vi "Core.vi"(8 "error in (no error)":errorcluster, 10 "Actor in":refnum<class "Actor.lvclass">, 11 "Reorder Driver Aliases Msg in":refnum<class "Reorder Driver Aliases Msg.lvclass">) -> (0 "error out":errorcluster, 1 "Data":refnum<class "Data.lvclass">, 2 "Actor out":refnum<class "Actor.lvclass">, 3 "Reorder Driver Aliases Msg out":refnum<class "Reorder Driver Aliases Msg.lvclass">)   [LabVIEW 2020, in "Instrument Handler.lvlib" / "Reorder Driver Aliases Msg.lvclass"]
doc: "Core of the Reponse Msg. Put the active code here.\n\nThis implementation reorders Alias' on the Instrument Handler. On a succesfull operation a TRUE is returned in a generic Boolean data class."
uses:
  Reorder Driver Aliases Msg.lvclass
  PPL/HDH.Data.Generic.lvlibp/Data.lvclass
  PPL/HDH.Actor Framework.Core.Actor.lvlibp/1abvi3w/vi.lib/ActorFramework/Actor/Actor.lvclass
  Instrument Handler/Instrument Handler.lvclass
  C:/Current projects/WS/PPL/HDH.Actor Framework.Core.Actor.lvlibp/1abvi3w/vi.lib/ActorFramework/Actor/Actor.lvclass
  Reorder Driver Aliases Msg.lvclass/Reorder Driver Aliases Msg.ctl
  PPL/HDH.Data.Generic.lvlibp/Generic Data/Boolean/Boolean.lvclass
  C:/Current projects/WS/PPL/HDH.Data.Generic.lvlibp/Data.lvclass
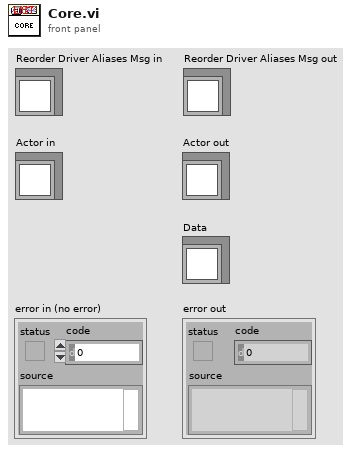
[diagram p1: front panel]
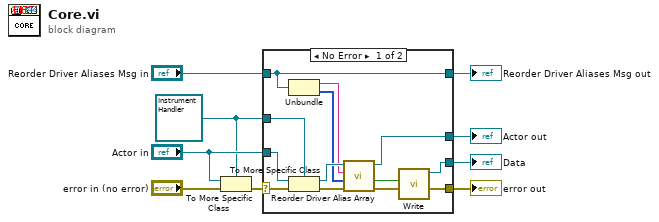
[diagram p0: block diagram]
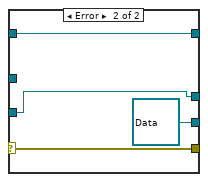
[diagram p2: hidden frame]
diagram:
  w5 = refnum<class "Instrument Handler.lvclass"> refnum ("Instrument Handler.lvlib:Instrument Handler.lvclass")
  n1 = To More Specific Class(target class=w5, reference="Actor in", error in="error in (no error)") -> (error out=w8:errorcluster)  [unwired: 1 out]
  n2 = case shown="No Error" w8 {
    selector: w8 -> [w21 w25]
    tunnel: [w10 w25] -> w7
    tunnel: [w13 w24] -> w4
    tunnel: "Actor in" -> [w20 w24]
    tunnel: w5 -> [w19 _]
    tunnel: [w11 refnum<class "Data.lvclass"> refnum ("Data")] -> w3
    tunnel: [w16 w22] -> w1
    tunnel: "Reorder Driver Aliases Msg in" -> [w16 w22]
    frame No Error {
      n3 = Unbundle(w16) -> (w15:string, w14:u32[])
      n4 = To More Specific Class(target class=w19, reference=w20, error in=w21) -> (specific class reference=w18:refnum<class "Instrument Handler.lvclass">, error out=w17:errorcluster)
      n5 = call "Reorder Driver Alias Array.vi"("error in (no error)"=w17, "New indices"=w14, "Driver Name"=w15, "Instrument Handler in"=w18) -> ("error out"=w10:errorcluster, "Success?"=w12:bool, "Instrument Handler out"=w13:refnum<class "Instrument Handler.lvclass">)  [unwired: 5 in]
      n6 = call "Write.vi"("Boolean"=w12) -> ("Boolean out"=w11:refnum<class "Boolean.lvclass">)  [unwired: 10 in]
    }
    frame Error {
    }
  }
  "error out" <- w7
  "Actor out" <- w4
  "Data" <- w3
  "Reorder Driver Aliases Msg out" <- w1
